vi "7HP_Convert serial string to Eng vals.vi"(0 "Serial buffer string (excluding FrameChar)":string) -> (3 "Pressures":sgl[][](graph), 4 "Atmospheric pressure (mbar)":sgl, 6 "External thermistor temperature (deg C)":sgl, 8 "Env. sensor die temperature (deg C)":sgl, 10 "Relative humidity (%)":sgl, 13 "All vals":sgl[](array[numeric]), 14 "Gyration vector (deg / s)":sgl[](array[numeric]), 15 "Acceleration vector (g)":sgl[](array[numeric]))   [LabVIEW 2020]
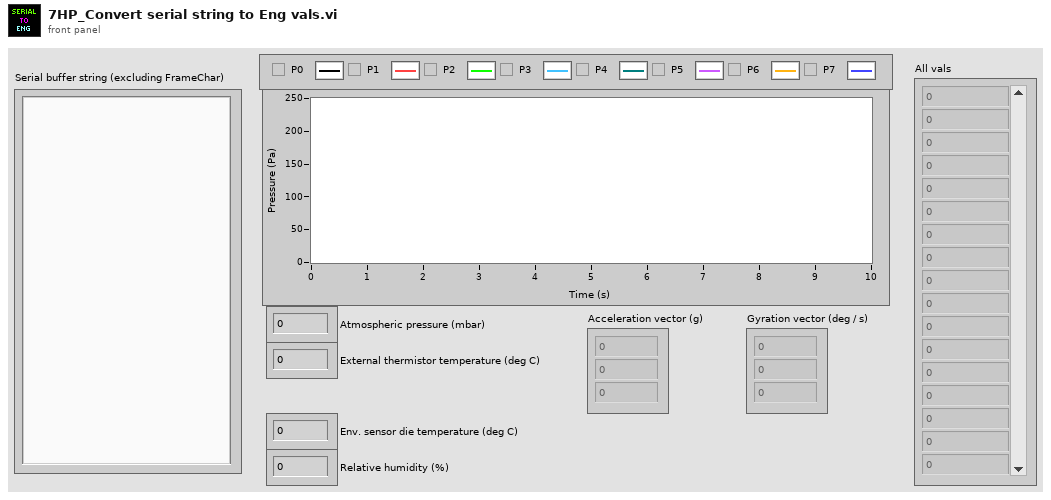
[diagram p1: front panel]
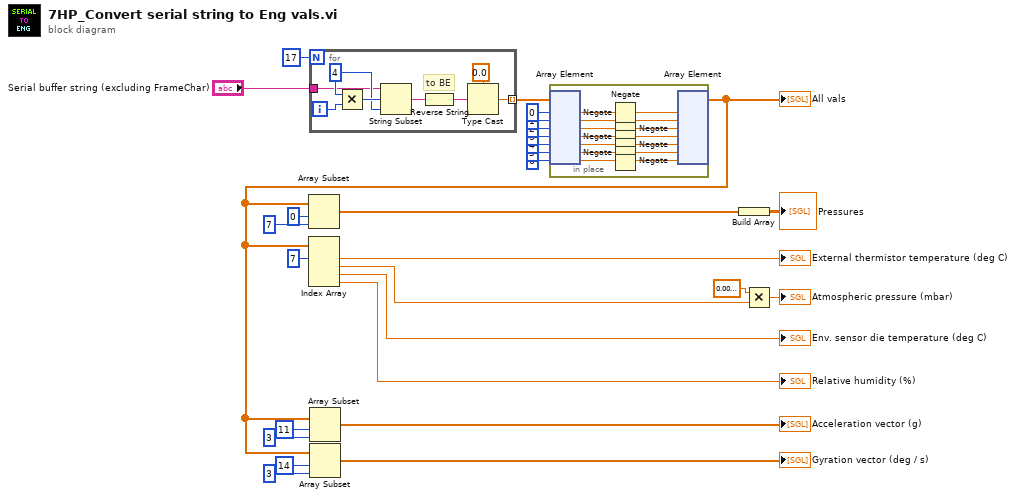
[diagram p0: block diagram]
diagram:
  n1 = for {
    N: 17 -> [_]
    tunnel: [w30] -> w25 mode=indexing
    tunnel: "Serial buffer string (excluding FrameChar)" -> [w29]
    i -> [w36]
    w34 = 4 ("x")
    # "to BE"
    n2 = Multiply(x=w34, y=w36) -> (x*y=w35:i32)
    n3 = String Subset(string=w29, offset (0)=w35, length (rest)=w34) -> (substring=w33:string)
    n4 = Reverse String(1:w33) -> (0:w32:string)
    n5 = Type Cast(type=sgl 0.0 ("byte count"), x=w32) -> (*(type *) &x=w30:sgl)
  }
  n6 = in-place {
    n7 = in-place-array #1(w25, 0, 1, 2, 3, 4, 5, 6) -> (w50:sgl, w49:sgl, w46:sgl, w45:sgl, w44:sgl, w38:sgl, w43:sgl)
    n8 = Negate(x=w50) -> (-x=w48:sgl)
    n9 = Negate(x=w49) -> (-x=w47:sgl)
    n10 = Negate(x=w46) -> (-x=w42:sgl)
    n11 = Negate(x=w45) -> (-x=w41:sgl)
    n12 = Negate(x=w44) -> (-x=w40:sgl)
    n13 = Negate(x=w38) -> (-x=w37:sgl)
    n14 = Negate(x=w43) -> (-x=w39:sgl)
    n15 = in-place-array #1(w48, w47, w42, w41, w40, w37, w39) -> (w1:sgl[])  [unwired: 7 out]
  }
  "All vals" <- w1
  n16 = Array Subset(array=w1, index=0, length=7) -> (w7:sgl[])
  n17 = Index Array(array=w1, index #1=7 ("index")) -> (element #1=→"External thermistor temperature (deg C)":sgl, element #2=w4:sgl, element #3=→"Env. sensor die temperature (deg C)":sgl, element #4=→"Relative humidity (%)":sgl)  [unwired: 3 in]
  n18 = Array Subset(array=w1, index=11, length=3) -> (→"Acceleration vector (g)":sgl[])
  n19 = Array Subset(array=w1, index=14, length=3) -> (→"Gyration vector (deg / s)":sgl[])
  n20 = Build Array(w7) -> (→"Pressures":sgl[][])
  n21 = Multiply(x=sgl 0.01, y=w4) -> (x*y=→"Atmospheric pressure (mbar)":sgl)
